vi "Config File Writer (VI Ref).vi"(0 "Append to file? (F)":bool, 4 "Parent Label":string, 5 "Parent Class":string, 6 "Close Config File? (T)":bool=TRUE, 7 "This VI":refnum<vi>, 8 "Only Enabled? (F)":bool, 9 "Only Visible? (T)":bool=TRUE, 11 "Config File Path":path=path "C:/Users/guillaume/Desktop") -> (3 "Ref Config File Out":T1)   [LabVIEW 2009]
uses:
  <vilib>/Utility/config.llb/Config Data RefNum.ctl
  <vilib>/Utility/config.llb/NI_LVConfig.lvlib
panel:
  # "Guillaume Plateau - Dec. 9, 2009\nyguig2@yahoo.fr - Version 3.0"
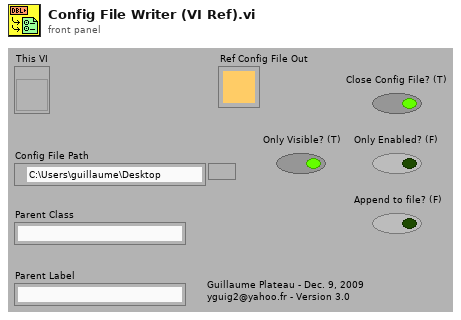
[diagram p1: front panel]
types:
  T1 = typedef "NI_LVConfig.lvlib/Config Data RefNum.ctl" = refnum<k1>
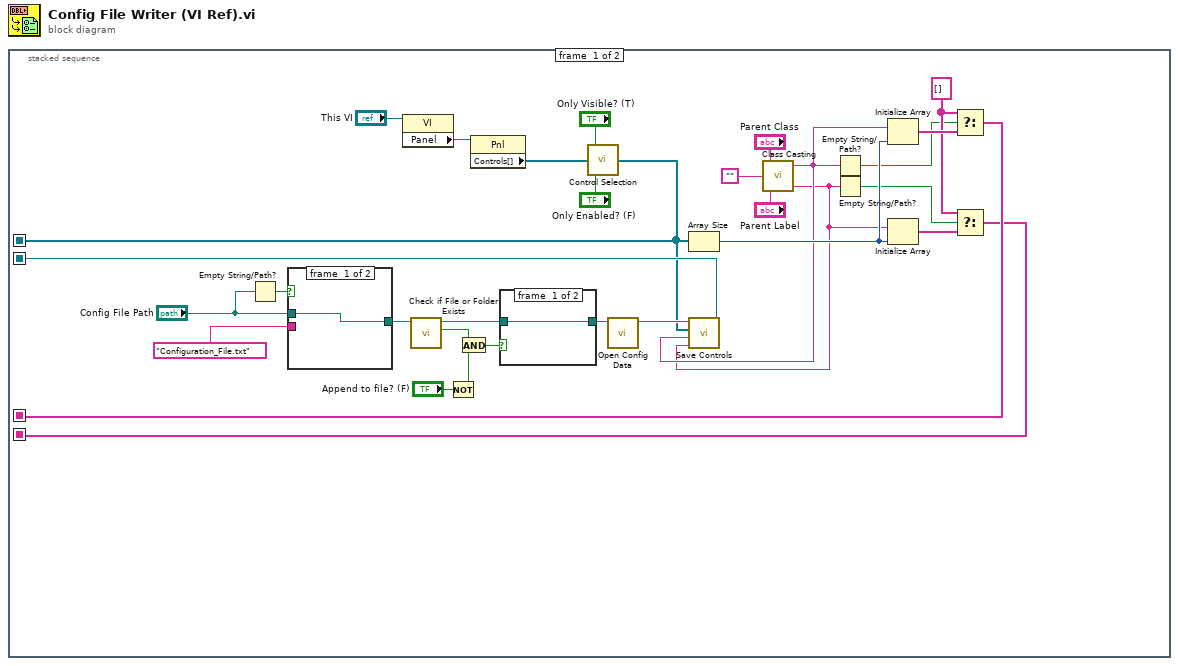
[diagram p0: block diagram]
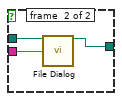
[diagram p2: hidden frame]
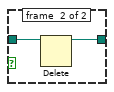
[diagram p3: hidden frame]
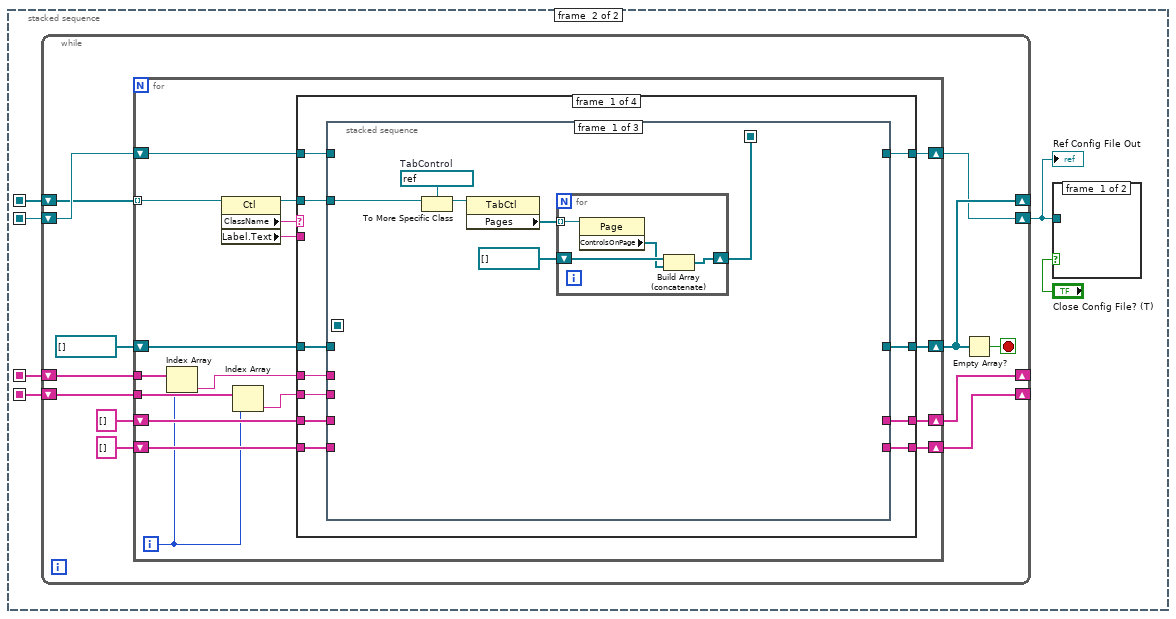
[diagram p4: hidden frame]
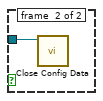
[diagram p5: hidden frame]
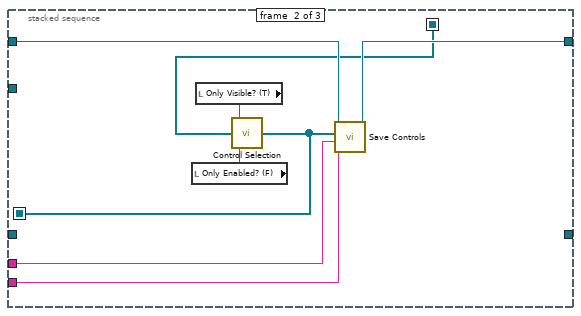
[diagram p6: hidden frame]
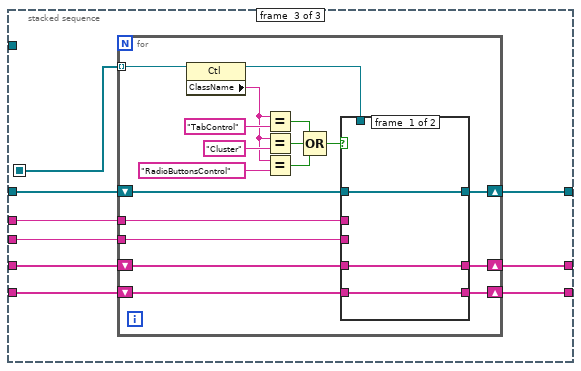
[diagram p7: hidden frame]
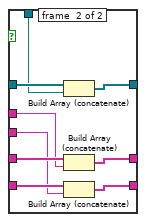
[diagram p8: hidden frame]
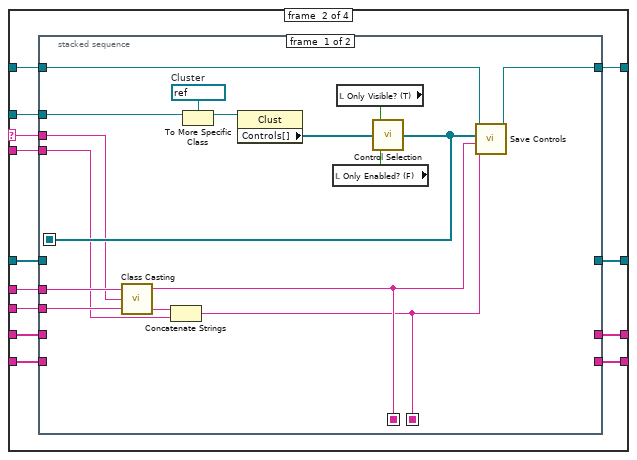
[diagram p9: hidden frame]
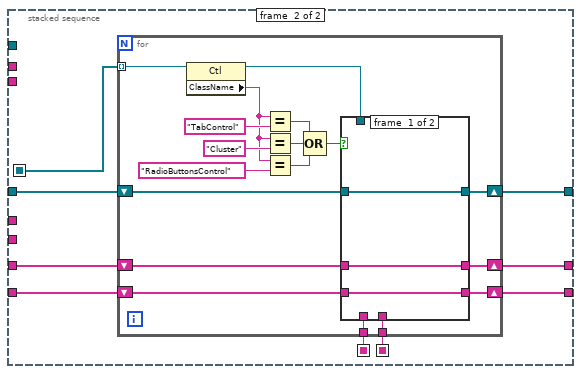
[diagram p10: hidden frame]
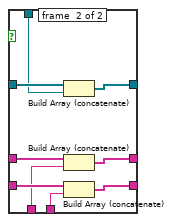
[diagram p11: hidden frame]
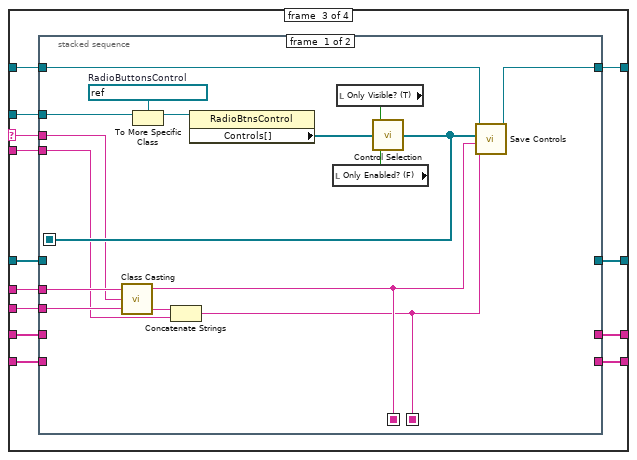
[diagram p12: hidden frame]
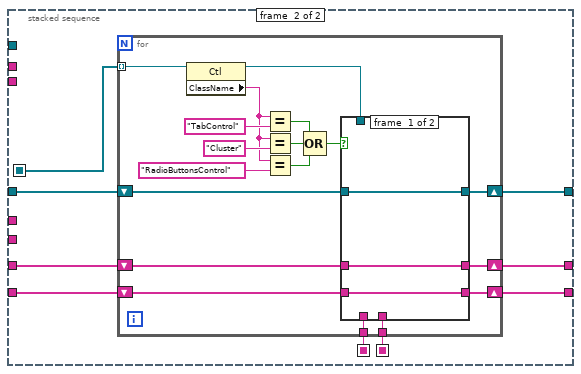
[diagram p13: hidden frame]
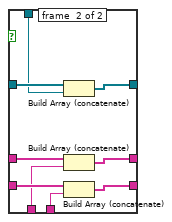
[diagram p14: hidden frame]
diagram:
  n1 = stacked-sequence {
    seq-local: [w17 _] -> [_ w44]
    seq-local: [w23 _] -> [_ w43]
    seq-local: [w10 _] -> [_ w40]
    seq-local: [w9 _] -> [_ w39]
    frame #0 {
      w13 = string[] [] ("t")
      n2 = Empty String/Path?(string/path="Config File Path") -> (empty?=w6:bool)
      n3 = case shown="True" w6 {
        tunnel: "Config File Path" -> [w32 w35]
        tunnel: "Configuration_File.txt" ("name or relative path") -> [_ w34]
        tunnel: [w32 w33] -> w25
        frame #0 {
        }
        frame #1 {
          n4 = call "File Dialog"("start path"=w35, "default name"=w34) -> ("selected path"=w33:path)  [unwired: 5 in, 8 out]
        }
      }
      n5 = property class="VI"(reference="This VI") -> ("Panel"=w30:refnum<vi>)  [unwired: 1 in, 2 out]
      n6 = call <vilib>:"Check if File or Folder Exists.vi"("path"=w25) -> ("file or folder exists?"=w5:bool, "dup path"=w31:path)  [unwired: 1 in, 8 out]
      n7 = Not(x="Append to file? (F)") -> (.not. x?=w1:bool)
      n8 = And(x=w5, y=w1) -> (x .and. y?=w4:bool)
      n9 = property class="Pnl"(reference=w30) -> ("Controls[]"=w2:refnum<vi>[])  [unwired: 1 in, 2 out]
      n10 = case shown="True" w4 {
        tunnel: w31 -> [w36 w38]
        tunnel: [w36 w37] -> w27
        frame #0 {
        }
        frame #1 {
          n11 = Delete(path (use dialog)=w38) -> (deleted path=w37:path)  [unwired: 1 in, 5 out]
        }
      }
      n12 = call "Control Selection.vi"("Only Enabled? (F)"="Only Enabled? (F)", "Controls In[]"=w2, "Only Visible? (T)"="Only Visible? (T)") -> ("Controls Out[]"=w17:refnum<vi>[])  [unwired: 1 in, 1 out]
      n13 = call <vilib>:"Open Config Data.vi"("configuration file path"=w27) -> ("refnum"=w28:T1)  [unwired: 8 in, 2 out]
      n14 = Array Size(array=w17) -> (size(s)=w16:i32)
      n15 = call "Class Casting.vi"("Parent Label"="Parent Label", "Control Class"="", "Parent Class"="Parent Class") -> ("Add-on Label"=w11:string, "Class"=w12:string)  [unwired: 1 out]
      n16 = call "Save Controls.vi"("Parent Label"=w11, "Parent Class"=w12, "Controls[]"=w17, "Ref Config File In"=w28) -> ("Ref Config File Out"=w23:T1)  [unwired: 7 out]
      n17 = Empty String/Path?(string/path=w12) -> (empty?=w8:bool)
      n18 = Empty String/Path?(string/path=w11) -> (empty?=w7:bool)
      n19 = Initialize Array(w12, w16) -> (w15:string[])
      n20 = Initialize Array(w11, w16) -> (w14:string[])
      n21 = Select(t=w13, s=w8, f=w15) -> (s? t:f=w10:string[])
      n22 = Select(t=w13, s=w7, f=w14) -> (s? t:f=w9:string[])
    }
    frame #1 {
      n23 = while {
        shift-right: [w57] -> _
        shift-left: w44 -> [w46]
        shift-right: [w55] -> w41
        shift-left: w43 -> [w56]
        shift-right: [w48] -> _
        shift-left: w40 -> [w52]
        shift-right: [w47] -> _
        shift-left: w39 -> [w51]
        stop <- w53 stop-if-true
        n24 = for {
          tunnel: w46 -> [w67] mode=indexing
          shift-right: [w71] -> w57
          shift-left: refnum<vi>[] [] -> [w72]
          shift-right: [w68] -> w55
          shift-left: w56 -> [w69]
          tunnel: w52 -> [w62]
          tunnel: w51 -> [w61]
          shift-right: [w64] -> w48
          shift-left: string[] [] -> [w66]
          shift-right: [w63] -> w47
          shift-left: string[] [] -> [w65]
          i -> [w60]
          n25 = Index Array(array=w62, index=w60) -> (element=w59:string)
          n26 = property class="Ctl"(reference=w67) -> (reference out=w73:refnum<vi>, "ClassName"=w74:string, "Label.Text"=w70:string)  [unwired: 1 in, 1 out]
          n27 = Index Array(array=w61, index=w60) -> (element=w58:string)
          n28 = case shown="\"TabControl\"" w74 {
            selector: w74 -> [_ w152 w221 _]
            tunnel: w73 -> [w85 w155 w222 _]
            tunnel: w72 -> [w82 w150 w219 w282]
            tunnel: [w81 w149 w213 w282] -> w71
            tunnel: w70 -> [_ w151 w220 _]
            tunnel: w69 -> [w84 w154 w223 w281]
            tunnel: [w83 w153 w214 w281] -> w68
            tunnel: w59 -> [w80 w148 w218 _]
            tunnel: w58 -> [w79 w147 w217 _]
            tunnel: w66 -> [w78 w144 w216 w280]
            tunnel: w65 -> [w77 w143 w215 w279]
            tunnel: [w76 w146 w212 w280] -> w64
            tunnel: [w75 w145 w211 w279] -> w63
            frame #0 {
              n29 = stacked-sequence {
                seq-local: [_ w98 _] -> [_ _ w112]
                seq-local: [w86 _ _] -> [_ w99 _]
                tunnel: w85 -> [w90 _ _]
                tunnel: w84 -> [_ w103 _]
                tunnel: [_ w102 _] -> w83
                tunnel: w82 -> [_ _ w111]
                tunnel: [_ _ w110] -> w81
                tunnel: w80 -> [_ w97 w105]
                tunnel: w79 -> [_ w96 w104]
                tunnel: w78 -> [_ _ w109]
                tunnel: w77 -> [_ _ w108]
                tunnel: [_ _ w107] -> w76
                tunnel: [_ _ w106] -> w75
                frame #0 {
                  w91 = refnum<vi> refnum  # TabControl
                  n30 = To More Specific Class(target class=w91, reference=w90) -> (specific class reference=w89:refnum<vi>)  [unwired: 1 in, 1 out]
                  n31 = property class="TabCtl"(reference=w89) -> ("Pages"=w88:refnum<vi>[])  [unwired: 1 in, 2 out]
                  n32 = for {
                    tunnel: w88 -> [w95] mode=indexing
                    shift-right: [w94] -> w86
                    shift-left: refnum<vi>[] [] -> [w93]
                    n33 = property class="Page"(reference=w95) -> ("ControlsOnPage"=w92:refnum<vi>[])  [unwired: 1 in, 2 out]
                    n34 = Build Array (concatenate)(w93, w92) -> (w94:refnum<vi>[])
                  }
                }
                frame #1 {
                  n35 = local read "Only Enabled? (F)"() -> (w100:bool)
                  n36 = local read "Only Visible? (T)"() -> (w101:bool)
                  n37 = call "Control Selection.vi"("Only Enabled? (F)"=w100, "Controls In[]"=w99, "Only Visible? (T)"=w101) -> ("Controls Out[]"=w98:refnum<vi>[])  [unwired: 2 out]
                  n38 = call "Save Controls.vi"("Parent Label"=w96, "Parent Class"=w97, "Controls[]"=w98, "Ref Config File In"=w103) -> ("Ref Config File Out"=w102:T1)  [unwired: 7 out]
                }
                frame #2 {
                  n39 = for {
                    tunnel: w112 -> [w130] mode=indexing
                    shift-right: [w120] -> w110
                    shift-left: w111 -> [w121]
                    shift-right: [w116] -> w107
                    shift-left: w109 -> [w119]
                    shift-right: [w115] -> w106
                    shift-left: w108 -> [w118]
                    tunnel: w105 -> [w114]
                    tunnel: w104 -> [w113]
                    n40 = property class="Ctl"(reference=w130) -> (reference out=w117:refnum<vi>, "ClassName"=w123:string)  [unwired: 1 in, 1 out]
                    n41 = Equal?(x=w123, y="TabControl") -> (x = y?=w126:bool)
                    n42 = Equal?(x=w123, y="Cluster") -> (x = y?=w125:bool)
                    n43 = Equal?(x=w123, y="RadioButtonsControl") -> (x = y?=w124:bool)
                    n44 = Compound Arithmetic op=OR(w126, w125, w124) -> (w122:bool)
                    n45 = case shown="True" w122 {
                      tunnel: w121 -> [w133 w142]
                      tunnel: w117 -> [_ w138]
                      tunnel: [w133 w141] -> w120
                      tunnel: w119 -> [w132 w140]
                      tunnel: w118 -> [w131 w139]
                      tunnel: [w132 w137] -> w116
                      tunnel: [w131 w136] -> w115
                      tunnel: w114 -> [_ w135]
                      tunnel: w113 -> [_ w134]
                      frame #0 {
                      }
                      frame #1 {
                        n46 = Build Array (concatenate)(w142, w138) -> (w141:refnum<vi>[])
                        n47 = Build Array (concatenate)(w140, w135) -> (w137:string[])
                        n48 = Build Array (concatenate)(w139, w134) -> (w136:string[])
                      }
                    }
                  }
                }
              }
            }
            frame #1 {
              n49 = stacked-sequence {
                seq-local: [w163 _] -> [_ w180]
                seq-local: [w157 _] -> [_ w173]
                seq-local: [w156 _] -> [_ w172]
                tunnel: w155 -> [w169 _]
                tunnel: w150 -> [_ w174]
                tunnel: [_ w179] -> w149
                tunnel: w154 -> [w165 _]
                tunnel: [w164 _] -> w153
                tunnel: w152 -> [w160 _]
                tunnel: w151 -> [w158 _]
                tunnel: w148 -> [w162 _]
                tunnel: w147 -> [w161 _]
                tunnel: [_ w178] -> w146
                tunnel: [_ w177] -> w145
                tunnel: w144 -> [_ w176]
                tunnel: w143 -> [_ w175]
                frame #0 {
                  w171 = refnum<vi> refnum  # Cluster
                  n50 = call "Class Casting.vi"("Parent Label"=w161, "Control Class"=w160, "Parent Class"=w162) -> ("Add-on Label"=w159:string, "Class"=w157:string)  [unwired: 1 out]
                  n51 = Concatenate Strings(w159, w158) -> (w156:string)
                  n52 = To More Specific Class(target class=w171, reference=w169) -> (specific class reference=w170:refnum<vi>)  [unwired: 1 in, 1 out]
                  n53 = property class="Clust"(reference=w170) -> ("Controls[]"=w166:refnum<vi>[])  [unwired: 1 in, 2 out]
                  n54 = local read "Only Enabled? (F)"() -> (w167:bool)
                  n55 = local read "Only Visible? (T)"() -> (w168:bool)
                  n56 = call "Control Selection.vi"("Only Enabled? (F)"=w167, "Controls In[]"=w166, "Only Visible? (T)"=w168) -> ("Controls Out[]"=w163:refnum<vi>[])  [unwired: 2 out]
                  n57 = call "Save Controls.vi"("Parent Label"=w156, "Parent Class"=w157, "Controls[]"=w163, "Ref Config File In"=w165) -> ("Ref Config File Out"=w164:T1)  [unwired: 7 out]
                }
                frame #1 {
                  n58 = for {
                    tunnel: w180 -> [w198] mode=indexing
                    shift-right: [w188] -> w179
                    shift-left: w174 -> [w189]
                    shift-right: [w184] -> w178
                    shift-left: w176 -> [w187]
                    shift-right: [w183] -> w177
                    shift-left: w175 -> [w186]
                    tunnel: w173 -> [w182]
                    tunnel: w172 -> [w181]
                    n59 = property class="Ctl"(reference=w198) -> (reference out=w185:refnum<vi>, "ClassName"=w191:string)  [unwired: 1 in, 1 out]
                    n60 = Equal?(x=w191, y="TabControl") -> (x = y?=w194:bool)
                    n61 = Equal?(x=w191, y="Cluster") -> (x = y?=w193:bool)
                    n62 = Equal?(x=w191, y="RadioButtonsControl") -> (x = y?=w192:bool)
                    n63 = Compound Arithmetic op=OR(w194, w193, w192) -> (w190:bool)
                    n64 = case shown="True" w190 {
                      tunnel: w189 -> [w201 w210]
                      tunnel: w185 -> [_ w206]
                      tunnel: [w201 w209] -> w188
                      tunnel: w187 -> [w200 w208]
                      tunnel: w186 -> [w199 w207]
                      tunnel: [w200 w205] -> w184
                      tunnel: [w199 w204] -> w183
                      tunnel: w182 -> [_ w203]
                      tunnel: w181 -> [_ w202]
                      frame #0 {
                      }
                      frame #1 {
                        n65 = Build Array (concatenate)(w210, w206) -> (w209:refnum<vi>[])
                        n66 = Build Array (concatenate)(w208, w203) -> (w205:string[])
                        n67 = Build Array (concatenate)(w207, w202) -> (w204:string[])
                      }
                    }
                  }
                }
              }
            }
            frame #2 {
              n68 = stacked-sequence {
                seq-local: [w235 _] -> [_ w248]
                seq-local: [w229 _] -> [_ w241]
                seq-local: [w228 _] -> [_ w240]
                tunnel: w222 -> [w225 _]
                tunnel: w219 -> [_ w242]
                tunnel: [_ w247] -> w213
                tunnel: w223 -> [w237 _]
                tunnel: [w236 _] -> w214
                tunnel: w221 -> [w232 _]
                tunnel: w220 -> [w230 _]
                tunnel: w218 -> [w234 _]
                tunnel: w217 -> [w233 _]
                tunnel: [_ w246] -> w212
                tunnel: [_ w245] -> w211
                tunnel: w216 -> [_ w244]
                tunnel: w215 -> [_ w243]
                frame #0 {
                  w227 = refnum<vi> refnum  # RadioButtonsControl
                  n69 = call "Class Casting.vi"("Parent Label"=w233, "Control Class"=w232, "Parent Class"=w234) -> ("Add-on Label"=w231:string, "Class"=w229:string)  [unwired: 1 out]
                  n70 = To More Specific Class(target class=w227, reference=w225) -> (specific class reference=w226:refnum<vi>)  [unwired: 1 in, 1 out]
                  n71 = Concatenate Strings(w231, w230) -> (w228:string)
                  n72 = property class="RadioBtnsControl"(reference=w226) -> ("Controls[]"=w224:refnum<vi>[])  [unwired: 1 in, 2 out]
                  n73 = local read "Only Enabled? (F)"() -> (w238:bool)
                  n74 = local read "Only Visible? (T)"() -> (w239:bool)
                  n75 = call "Control Selection.vi"("Only Enabled? (F)"=w238, "Controls In[]"=w224, "Only Visible? (T)"=w239) -> ("Controls Out[]"=w235:refnum<vi>[])  [unwired: 2 out]
                  n76 = call "Save Controls.vi"("Parent Label"=w228, "Parent Class"=w229, "Controls[]"=w235, "Ref Config File In"=w237) -> ("Ref Config File Out"=w236:T1)  [unwired: 7 out]
                }
                frame #1 {
                  n77 = for {
                    tunnel: w248 -> [w266] mode=indexing
                    shift-right: [w256] -> w247
                    shift-left: w242 -> [w257]
                    shift-right: [w252] -> w246
                    shift-left: w244 -> [w255]
                    shift-right: [w251] -> w245
                    shift-left: w243 -> [w254]
                    tunnel: w241 -> [w250]
                    tunnel: w240 -> [w249]
                    n78 = property class="Ctl"(reference=w266) -> (reference out=w253:refnum<vi>, "ClassName"=w259:string)  [unwired: 1 in, 1 out]
                    n79 = Equal?(x=w259, y="TabControl") -> (x = y?=w262:bool)
                    n80 = Equal?(x=w259, y="Cluster") -> (x = y?=w261:bool)
                    n81 = Equal?(x=w259, y="RadioButtonsControl") -> (x = y?=w260:bool)
                    n82 = Compound Arithmetic op=OR(w262, w261, w260) -> (w258:bool)
                    n83 = case shown="True" w258 {
                      tunnel: w257 -> [w269 w278]
                      tunnel: w253 -> [_ w274]
                      tunnel: [w269 w277] -> w256
                      tunnel: w255 -> [w268 w276]
                      tunnel: w254 -> [w267 w275]
                      tunnel: [w268 w273] -> w252
                      tunnel: [w267 w272] -> w251
                      tunnel: w250 -> [_ w271]
                      tunnel: w249 -> [_ w270]
                      frame #0 {
                      }
                      frame #1 {
                        n84 = Build Array (concatenate)(w278, w274) -> (w277:refnum<vi>[])
                        n85 = Build Array (concatenate)(w276, w271) -> (w273:string[])
                        n86 = Build Array (concatenate)(w275, w270) -> (w272:string[])
                      }
                    }
                  }
                }
              }
            }
            frame #3 {
            }
          }
        }
        n87 = Empty Array?(array=w57) -> (empty?=w53:bool)
      }
      "Ref Config File Out" <- w41
      n88 = case shown="True" "Close Config File? (T)" {
        tunnel: w41 -> [_ w45]
        frame #0 {
        }
        frame #1 {
          n89 = call <vilib>:"Close Config Data.vi"("refnum"=w45) -> ()  [unwired: 2 in, 9 out]
        }
      }
    }
  }
